vi "GetConfigInfo.vi"(5 "error in (no error)":errorcluster caption="错误输入（无错误）") -> (14 "串口配置":string[][](array[string]), 19 "error out":errorcluster)   [LabVIEW 2013]
uses:
  <vilib>/Utility/config.llb/Read Key (String).vi
  <vilib>/Utility/config.llb/NI_LVConfig.lvlib
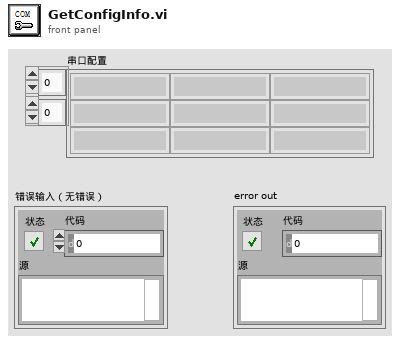
[diagram p1: front panel]
types:
  T1 = typedef "NI_LVConfig.lvlib/Config Data RefNum.ctl" = refnum<k1>
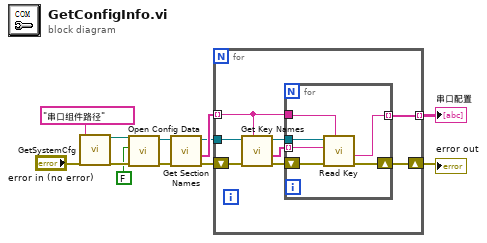
[diagram p0: block diagram]
diagram:
  n1 = call "GetSystemCfg.vi"("SystemCfg"="串口组件路径", "error in (no error)"="error in (no error)") -> ("Ini File Path"=w11:path, "error out"=w10:errorcluster)  [unwired: 16 in]
  n2 = call <vilib>:"Open Config Data.vi"("error in (no error)"=w10, "create file if necessary (T)"=FALSE, "configuration file path"=w11) -> ("error out"=w7:errorcluster, "refnum"=w8:T1)  [unwired: 6 in, 1 out]
  n3 = call <vilib>:"Get Section Names.vi"("error in (no error)"=w7, "refnum"=w8) -> ("error out"=w4:errorcluster, "section names"=w6:string[], "refnum out"=w5:T1)  [unwired: 7 in]
  n4 = for {
    tunnel: w6 -> [w17] mode=indexing
    tunnel: w5 -> [w19]
    shift-right: [w13] -> w1
    shift-left: w4 -> [w20]
    tunnel: [w16] -> w3 mode=indexing
    n5 = call <vilib>:"Get Key Names.vi"("section"=w17, "error in (no error)"=w20, "refnum"=w19) -> ("error out"=w14:errorcluster, "key names"=w18:string[], "refnum out"=w15:T1)  [unwired: 5 in, 1 out]
    n6 = for {
      tunnel: w18 -> [w25] mode=indexing
      tunnel: w17 -> [w26]
      tunnel: [w24] -> w16 mode=indexing
      tunnel: w15 -> [w23]
      shift-right: [w21] -> w13
      shift-left: w14 -> [w22]
      n7 = call-poly <vilib>:"Read Key.vi"("section"=w26, "error in (no error)"=w22, "key"=w25, "refnum"=w23) -> ("error out"=w21:errorcluster, "value"=w24:string)  [unwired: 4 in, 2 out]
    }
  }
  "串口配置" <- w3
  "error out" <- w1
